vi "User Interface Global.vi"(6 "data2":variant, 7 "command":T1=enum."Update UI", 8 "error in":errorcluster, 9 "data1":variant, 10 "action":T2, 11 "user interface":refnum<queue>) -> (0 "error out":errorcluster)   [LabVIEW 2011]
uses:
  Controls/User Interface Action.ctl
  User Interface Global Action.ctl
  Controls/User Interface Control.ctl
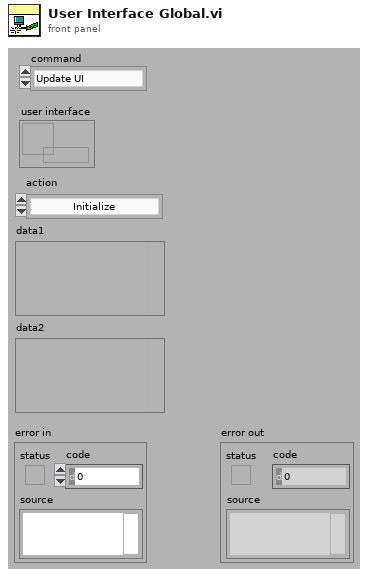
[diagram p1: front panel]
types:
  T1 = typedef "User Interface Global Action.ctl" = enum16{"Initialize", "Update UI", "Stop"}
  T2 = typedef "User Interface Action.ctl" = enum16{"Initialize", "Visibility Front Panel Controls", "Stop"}
  T3 = typedef "User Interface Control.ctl" = cluster{"action":T2, "data1":variant, "data2":variant}
  T4 = typedef "User Interface Queue Reference.ctl" = refnum<queue>
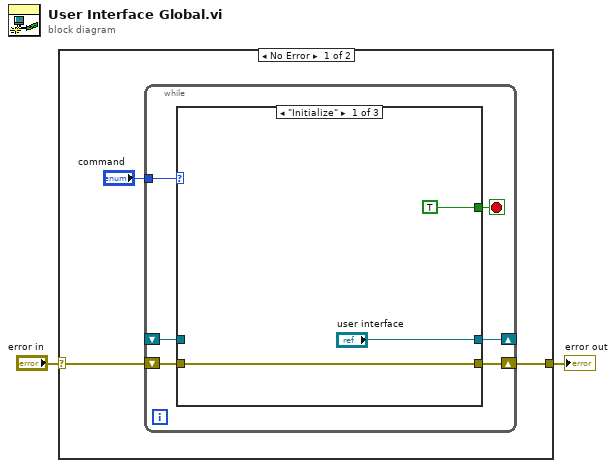
[diagram p0: block diagram]
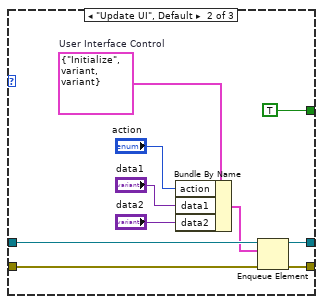
[diagram p2: hidden frame]
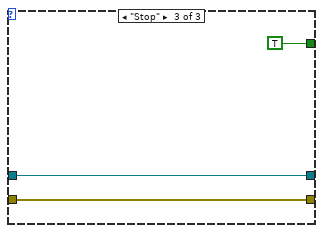
[diagram p3: hidden frame]
diagram:
  n1 = case shown="No Error" "error in" {
    selector: "error in" -> [w5 w28]
    tunnel: [w4 w28] -> w1
    frame No Error {
      n2 = while {
        shift-right: [w9] -> w4
        shift-left: w5 -> [w10]
        tunnel: "command" -> [w8]
        shift-right: [w7] -> _
        shift-left: _ -> [w6]
        stop <- w11 stop-if-true
        n3 = case shown="\"Initialize\"" w8 {
          tunnel: [TRUE TRUE TRUE] -> w11
          tunnel: w10 -> [w13 w22 w27]
          tunnel: [w13 w21 w27] -> w9
          tunnel: ["user interface" w18 w25] -> w7
          tunnel: w6 -> [_ w20 w25]
          frame "Initialize" {
          }
          frame "Update UI", Default {
            w15 = T3 {"action"=enum."Initialize", "data1"=variant, "data2"=variant}  # User Interface Control
            n4 = Bundle By Name(cluster=w15, "action"="action", "data1"="data1", "data2"="data2") -> (w19:T3)
            n5 = Enqueue Element(queue=w20, element=w19, error in (no error)=w22) -> (queue out=w18:T4, error out=w21:errorcluster)  [unwired: 1 in, 1 out]
          }
          frame "Stop" {
          }
        }
      }
    }
    frame Error {
    }
  }
  "error out" <- w1
